vi "NI ARC full _ kyles.vi"() -> ()   [LabVIEW 2012]
uses:
  <vilib>/Platform/TimedLoop/XDataNode/timing_clust.ctl
  <vilib>/Platform/TimedLoop/XDataNode/nitl_modes.ctl
  <vilib>/Platform/TimedLoop/XDataNode/wakeup.ctl
  <vilib>/FPGAPlugInAG/sbRIO-9636/niLvFpga_Open_sbRIO-9636.vi
  <vilib>/rvi/interface/common/dynamic/niFpgaDynamicAddResources.vi
  <vilib>/Utility/error.llb/Error Cluster From Error Code.vi
  <vilib>/rvi/errors/niLvFpgaAdjustHostInterfaceError.vi
  Globals.vi
  <vilib>/FPGAPlugInAG/Dynamic/niLvFpga_Close_Dynamic.vi
  <vilib>/rvi/interface/nirviOpenFPGA/nirviOpenFPGA.xnode
  FPGA Bitfiles/NIARC_FPGATarget_FPGACompile_e4XhunWUay0.lvbitx
  <vilib>/rvi/interface/nirviReadWriteControl/nirviReadWriteControl.xnode
  <vilib>/platform/TimedLoop/XDataNode/XDataNode.xnode
  <vilib>/rvi/interface/nirviCloseFPGA/nirviCloseFPGA.xnode
  NiFpgaLv.dll
  <vilib>/rvi/interface/Simulation/niFpgaSimulationCallBeginRW.vi
  <vilib>/Platform/TimedLoop/XDataNode/XDNodeRunTimeDep.lvlib
panel:
  in  "STOP":bool
  in  "stop":bool
  in  "Enable":bool
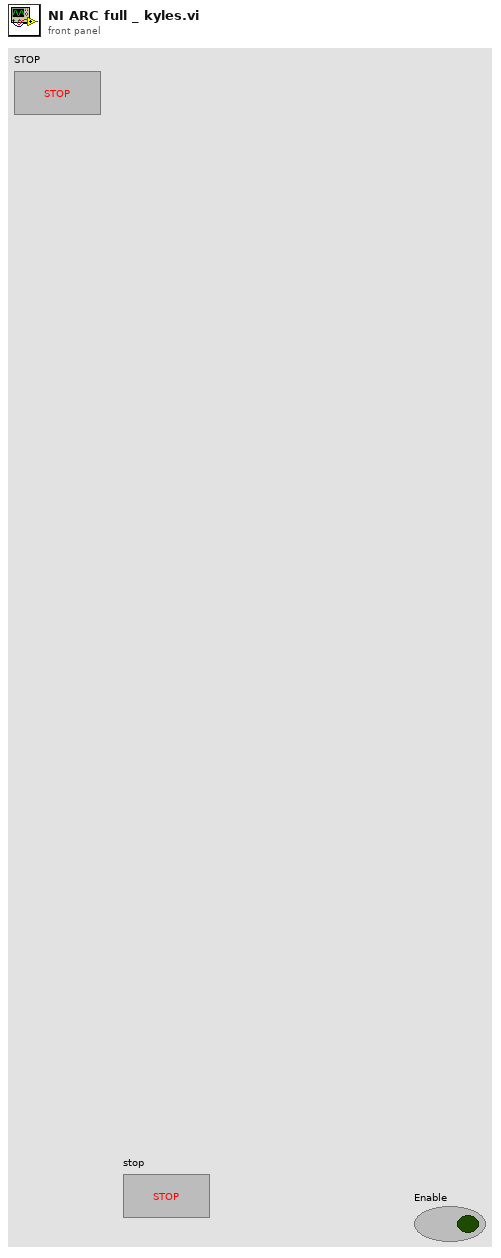
[diagram p1: front panel]
types:
  T1 = cluster{"m":fxp<+,17,2>, "b":fxp<+,15,-1>, "k":fxp<+,21,-4>}
  T2 = typedef "XDNodeRunTimeDep.lvlib/timing_clust.ctl" = cluster{"Expected End [f-1]":u64, "Actual End [f-1]":u64, "Finished Late? [f-1]":bool, "Expected End [i-1]":u64, "Actual End [i-1]":u64, "Finished Late? [i-1]":bool, "Expected Start [i]":u64, "Actual Start [i]":u64, "Expected Start [f]":u64, "Actual Start [f]":u64, "Source Name":string, "Structure Name":string, "Period":i64, "Deadline":i64, "Offset":i64, "Start":i64, "Priority":i32, "Timeout":i32, "Mode":T3, "Wakeup Reason":T4, "Error":errorcluster, "Source Type":string, "Secondary Source Type":string, "Global End Time":u64, "Global Start Time":u64, "Frame Duration":u64, "Iteration Duration":u64, "Assigned CPU":i32, "I/O Scan Engine Mode":u32}
  T3 = typedef "XDNodeRunTimeDep.lvlib/nitl_modes.ctl" = enum32{"No Change", "Process missed periods, maintain original phase", "Discard missed periods, maintain original phase", "Process missed periods, ignore original phase", "Discard missed periods, ignore original phase"}
  T4 = typedef "XDNodeRunTimeDep.lvlib/wakeup.ctl" = enum32{"Normal", "Aborted", "Asynchronous wakeup", "Timing source error", "Timed loop error", "Timeout"}
  T5 = cluster{"m":fxp<+,17,2>, "b":fxp<+,15,-1>, "k":fxp<+,21,-4>}[]
  T6 = cluster{"X Velocity (m/s)":dbl, "Y Velocity (m/s)":dbl, "Angular Velocity (rad/s)":dbl}
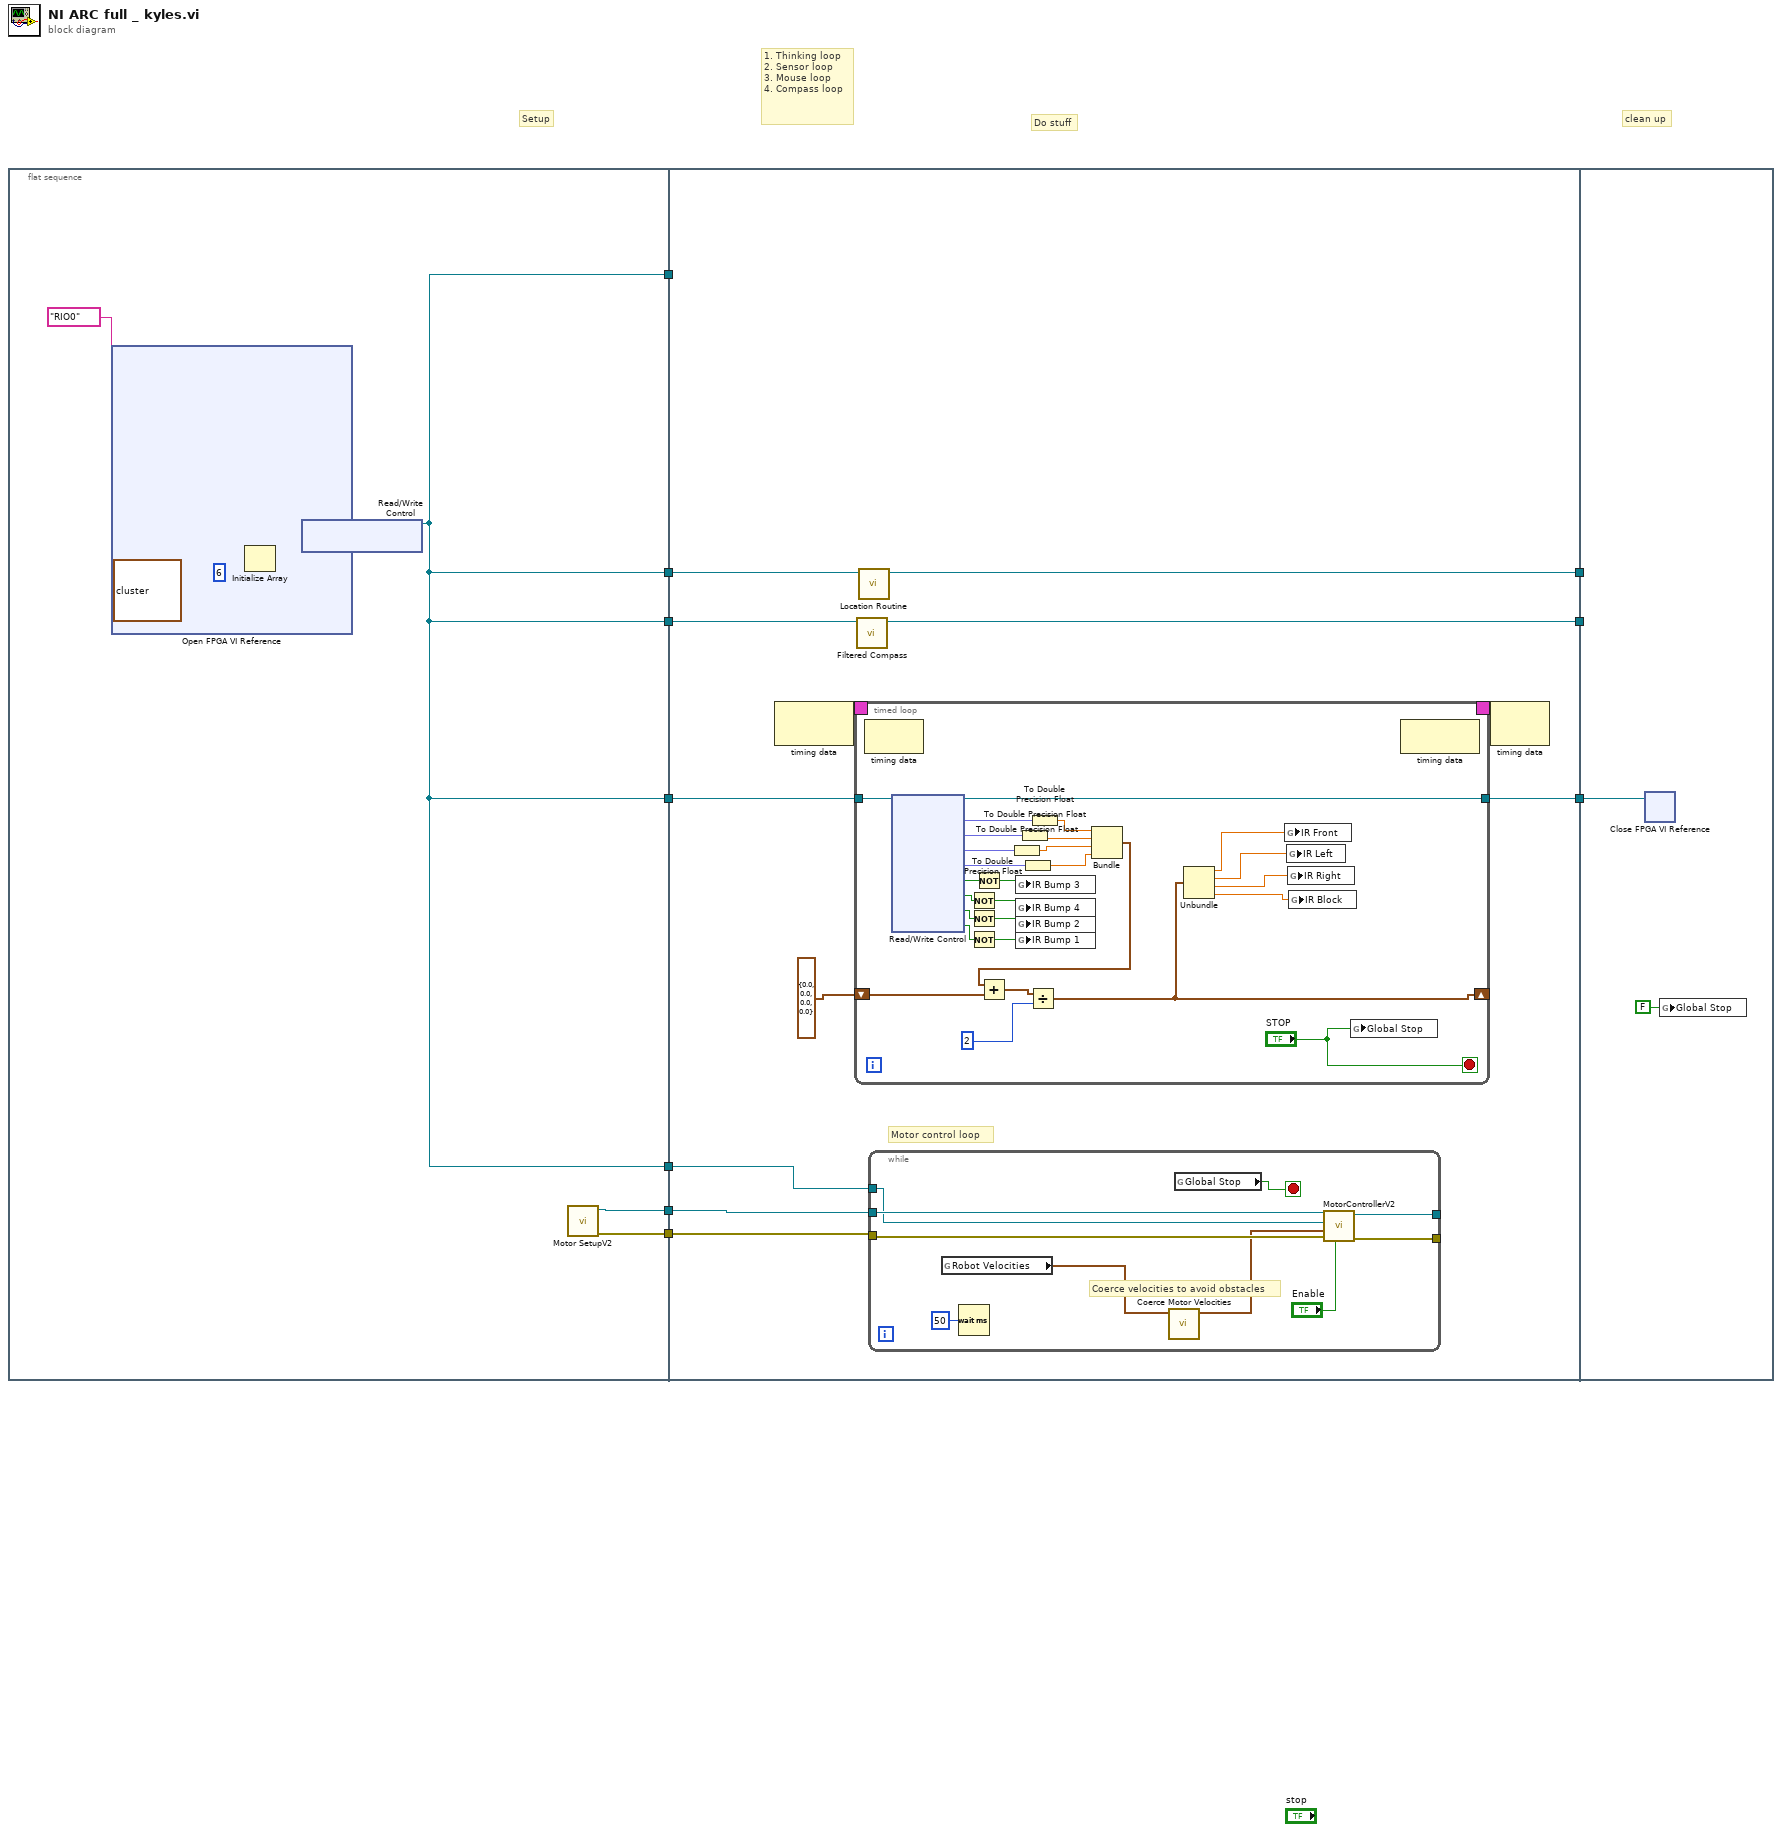
[diagram p0: block diagram]
diagram:
  # "clean up"
  # "Do stuff"
  # "Setup"
  # "1. Thinking loop\n2. Sensor loop\n3. Mouse loop\n4. Compass loop"
  n1 = flat-sequence {
    tunnel: [w18] -> w10
    tunnel: [w17] -> w9
    tunnel: [w11] -> w8
    tunnel: [w11] -> w7
    tunnel: [w11] -> w6
    tunnel: [w11] -> w4
    tunnel: [w11] -> w2
    tunnel: w10 -> [w29]
    tunnel: w9 -> [w30]
    tunnel: w8 -> [_]
    tunnel: w7 -> [w28]
    tunnel: w6 -> [w24]
    tunnel: [w23] -> w5
    tunnel: w4 -> [w22]
    tunnel: [w21] -> w3
    tunnel: w2 -> [w20]
    tunnel: [w19] -> w1
    tunnel: w5 -> [w74]
    tunnel: w3 -> [_]
    tunnel: w1 -> [_]
    frame #0 {
      n2 = xnode "Open FPGA VI Reference"("resource name"=tag "RIO0") -> ("FPGA VI Reference Out"=w15:refnum<k20>)  [unwired: 1 in, 1 out]
      n3 = Initialize Array(T1 {"m"=3.0281982421875, "b"=0.300506591796875, "k"=0.04309991002082825} ("Calibration Parameters"), 6 ("dimension size")) -> (w12:T5)
      n4 = xnode "Read/Write Control"("FPGA VI Reference In"=w15, "IR Calibration Array"=w12) -> ("FPGA VI Reference Out"=w11:refnum<k20>)  [unwired: 1 in, 1 out]
      n5 = call "Motor SetupV2.vi"() -> ("error out"=w17:errorcluster, "mecanum steering frame out"=w18:refnum<class "NI_Robotics_Mecanum Steering Frame.lvclass">)  [unwired: 10 in]
    }
    frame #1 {
      # "Motor control loop"
      n6 = node-c288() -> (w27:T2)  [unwired: 1 in]
      n7 = timed-loop {
        timing: w27 -> [_]
        timing-out: [_] -> w26
        tunnel: w24 -> [w58]
        shift-right: [w47] -> _
        shift-left: cluster{dbl, dbl, dbl, dbl} {0.0, 0.0, 0.0, 0.0} -> [w51]
        tunnel: [w43] -> w23
        stop <- "STOP" stop-if-true
        n8 = node-c288() -> ()  [unwired: 1 in, 1 out]
        n9 = xnode "Read/Write Control"("FPGA VI Reference In"=w58) -> ("FPGA VI Reference Out"=w43:refnum<k20>, "IR 0"=w57:fxp<+/-,24,5>, "IR 1"=w56:fxp<+/-,24,5>, "IR 2"=w55:fxp<+/-,24,5>, "IR 3"=w42:fxp<+/-,24,5>, "IR Bump 3"=w39:bool, "IR Bump 4"=w38:bool, "IR Bump 2"=w34:bool, "IR Bump 1"=w32:bool)  [unwired: 1 in, 1 out]
        n10 = Not(x=w38) -> (.not. x?=w36:bool)
        n11 = Not(x=w34) -> (.not. x?=w35:bool)
        n12 = Not(x=w32) -> (.not. x?=w33:bool)
        n13 = Not(x=w39) -> (.not. x?=w37:bool)
        n14 = To Double Precision Float(number=w55) -> (double precision float=w52:dbl)
        n15 = global write "Globals.vi" "IR Bump 3"(w37) -> ()
        n16 = global write "Globals.vi" "IR Bump 4"(w36) -> ()
        n17 = global write "Globals.vi" "IR Bump 2"(w35) -> ()
        n18 = global write "Globals.vi" "IR Bump 1"(w33) -> ()
        n19 = To Double Precision Float(number=w56) -> (double precision float=w53:dbl)
        n20 = To Double Precision Float(number=w42) -> (double precision float=w41:dbl)
        n21 = To Double Precision Float(number=w57) -> (double precision float=w54:dbl)
        n22 = Bundle(w54, w53, w52, w41) -> (w50:cluster{dbl, dbl, dbl, dbl})  [unwired: 1 in]
        n23 = Add(x=w50, y=w51) -> (x+y=w49:cluster{dbl, dbl, dbl, dbl})
        n24 = Divide(x=w49, y=2) -> (x/y=w47:cluster{dbl, dbl, dbl, dbl})
        n25 = Unbundle(w47) -> (w46:dbl, w45:dbl, w44:dbl, w40:dbl)
        n26 = global write "Globals.vi" "IR Front"(w46) -> ()
        n27 = global write "Globals.vi" "IR Left"(w45) -> ()
        n28 = global write "Globals.vi" "IR Right"(w44) -> ()
        n29 = global write "Globals.vi" "IR Block"(w40) -> ()
        n30 = global write "Globals.vi" "Global Stop"("STOP") -> ()
        n31 = node-c288() -> ()  [unwired: 1 in, 1 out]
      }
      n32 = call "Filtered Compass.vi"("FPGA Reference In"=w22) -> ("FPGA Reference Out"=w21:refnum<k20>)  [unwired: 10 in]
      n33 = call "Location Routine.vi"("Refnum in"=w20) -> ("Refnum out"=w19:refnum<k20>)  [unwired: 9 in, 1 out]
      n34 = while {
        tunnel: w29 -> [w72]
        tunnel: w30 -> [w71]
        tunnel: w28 -> [w66]
        tunnel: [w65] -> _
        tunnel: [w64] -> _
        stop <- w63 stop-if-true
        # "Coerce velocities to avoid obstacles"
        n35 = global read "Globals.vi" "Robot Velocities"() -> (w68:T6)
        n36 = Wait (ms)(milliseconds to wait=u32 50) -> ()  [unwired: 1 out]
        n37 = call "Coerce Motor Velocities.vi"("Robot Velocities in"=w68) -> ("Robot Velocities out"=w67:T6)  [unwired: 10 in]
        n38 = global read "Globals.vi" "Global Stop"() -> (w63:bool)
        n39 = call "MotorControllerV2.vi"("Enable"="Enable", "error in"=w71, "Robot Velocities"=w67, "FPGA VI Reference In"=w66, "mecanum steering frame in"=w72) -> ("error out"=w64:errorcluster, "steering frame out"=w65:refnum<class "NI_Robotics_Mecanum Steering Frame.lvclass">)  [unwired: 5 in]
      }
      n40 = node-c288(w26) -> ()  [unwired: 1 out]
    }
    frame #2 {
      n41 = xnode "Close FPGA VI Reference"("FPGA VI Reference In"=w74) -> ()  [unwired: 1 in, 1 out]
      n42 = global write "Globals.vi" "Global Stop"(FALSE ("Global Stop")) -> ()
    }
  }
